vi "Create IntelliSense Control.vi"(11 "error in":errorcluster) -> (4 "IntelliSense Control":refnum<class "IntelliSenseStringControl.lvclass">, 15 "error out":errorcluster)   [LabVIEW 2016, in "StringIntelliSense.lvlib" / "IntelliSenseStringControl.lvclass"]
uses:
  IntelliSenseStringControl.lvclass
  Typedefs/String Monitor Details.ctl
  IntelliSenseStringControl.lvclass/IntelliSenseStringControl.ctl
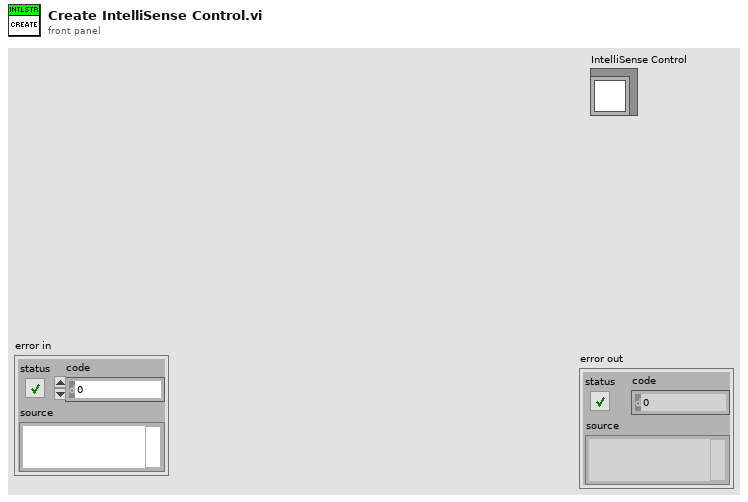
[diagram p1: front panel]
types:
  T1 = typedef "StringIntelliSense.lvlib/IntelliSenseStringControl.lvclass/String Monitor Details.ctl" = cluster{"Str ctrl Suggestion":string[], "Case Sensitive Suggestions?":bool, "Append User String to Suggestion?":bool, "Autofill Suggestion Choices?":bool}
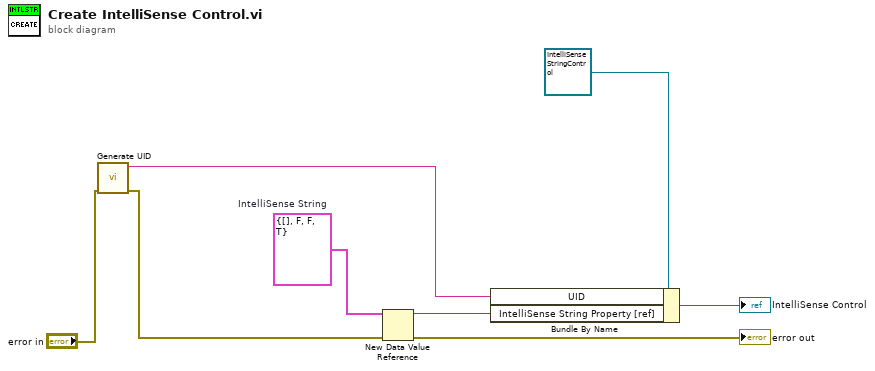
[diagram p0: block diagram]
diagram:
  w8 = T1 {"Str ctrl Suggestion"=[], "Case Sensitive Suggestions?"=FALSE, "Append User String to Suggestion?"=FALSE, "Autofill Suggestion Choices?"=TRUE}  # IntelliSense String
  n1 = call "Generate UID.vi"("Error In"="error in") -> ("error out"=w2:errorcluster, "GUID"=w3:string)  [unwired: 9 in]
  n2 = New Data Value Reference(data value=w8, error in=w2) -> (data value reference=w5:refnum<data-value>, error out=→"error out":errorcluster)
  n3 = Bundle By Name(cluster=refnum<class "IntelliSenseStringControl.lvclass"> refnum ("StringIntelliSense.lvlib:IntelliSense String"), "UID"=w3, "IntelliSense String Property [ref]"=w5) -> (→"IntelliSense Control":refnum<class "IntelliSenseStringControl.lvclass">)
